vi "Server UI.vi"(11 "LV Chat Server in":refnum<class "LV Chat Server.lvclass">) -> (3 "LV Chat Server":refnum<class "LV Chat Server.lvclass">)   [LabVIEW 2020, in "LV Chat Server.lvclass"]
uses:
  LV Chat Server.lvclass
  UI State.ctl
  Data Types/Message.ctl
  LV Chat Server.lvclass/LV Chat Server.ctl
  Events.ctl
  Stream-Simple-Msg/Endpoint/Endpoint.lvclass
  Log Event Data.ctl
panel:
  in  "Timestamps":bool
  out "Time Connected":dbl format="%<%m/%d %H:%M:%S>T"
  out "Connection":string
  out "Users Connected":i32
  in  "Kick User":bool
  out "Log":string
  in  "Users":i32(listbox)
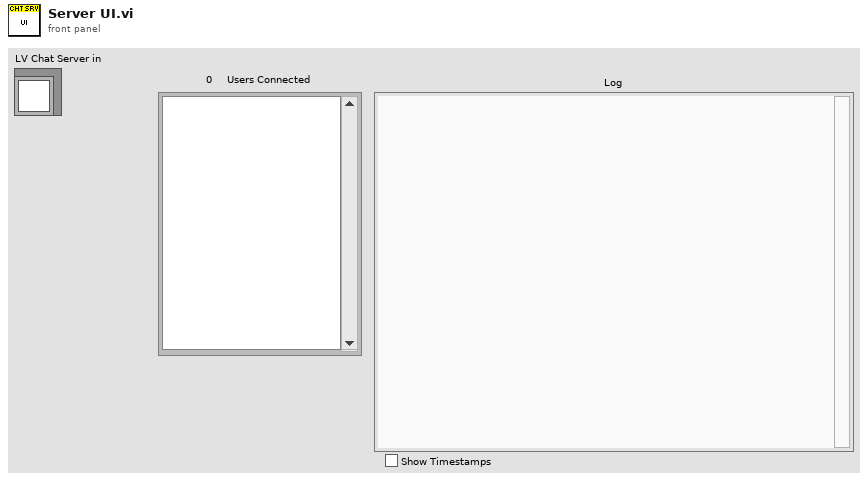
[diagram p1: front panel]
types:
  T1 = typedef "LV Chat Server.lvclass/UI State.ctl" = enum16{"Init", "Run", "Close"}
  T2 = typedef "Message.ctl" = cluster{"From":string, "Time":dbl, "Message":string}
  T3 = typedef "LV Chat Server.lvclass/Events.ctl" = cluster{"New Connection":refnum<user-event>, "Log":refnum<user-event>, "Refresh Log":refnum<user-event>, "Refresh Users":refnum<user-event>}
  T4 = typedef "LV Chat Server.lvclass/Ref Data.ctl" = cluster{"Endpoint Map":map{string, T5}, "User Map":map{string, string}}
  T5 = typedef "LV Chat Server.lvclass/User.ctl" = cluster{"Name":string, "IP":string, "Connected At":dbl, "Endpoint":refnum<class "Endpoint.lvclass">}
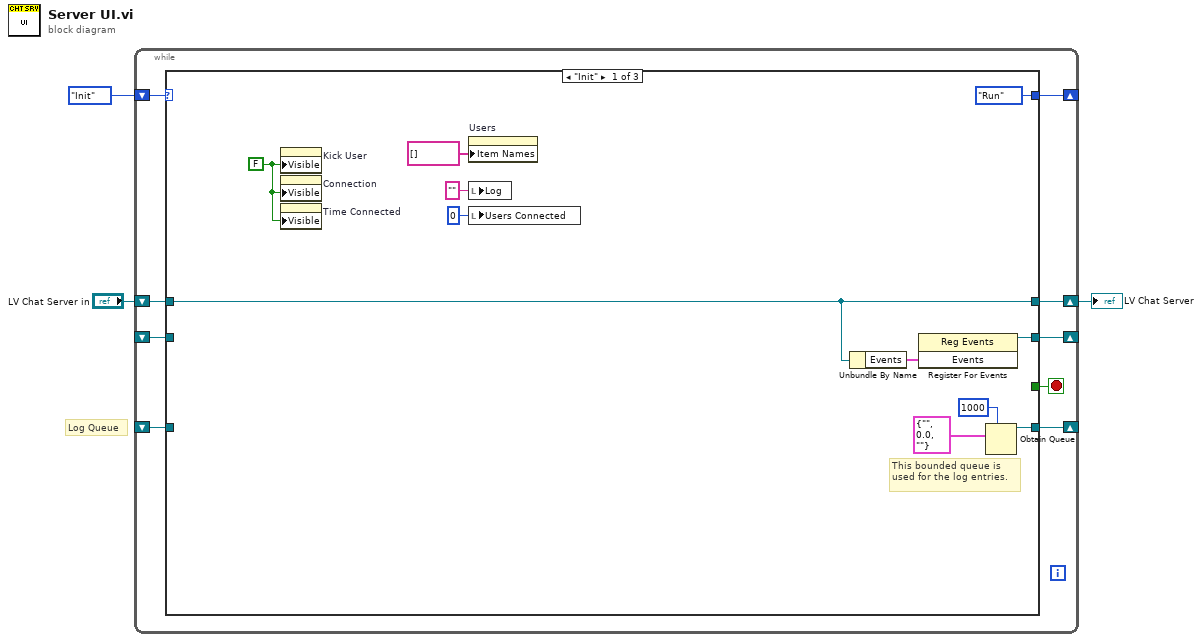
[diagram p0: block diagram]
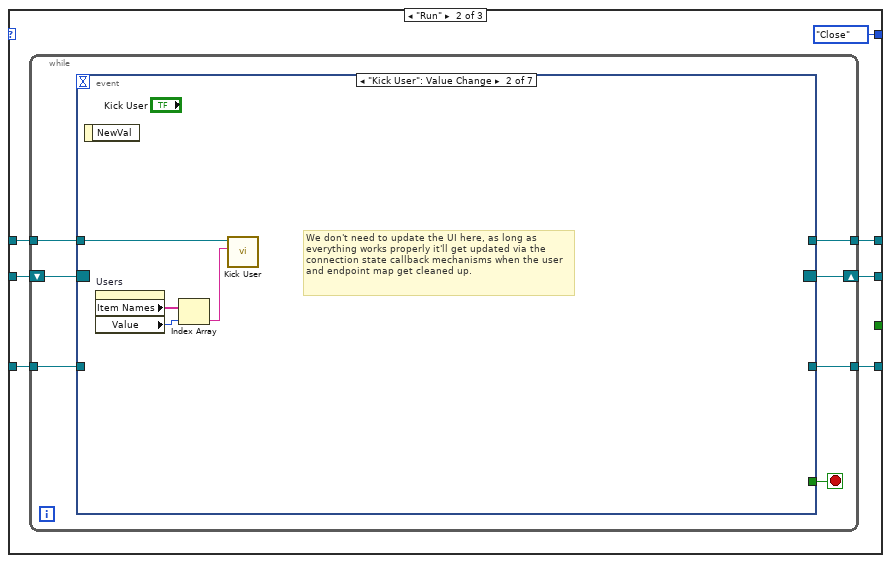
[diagram p2: hidden frame]
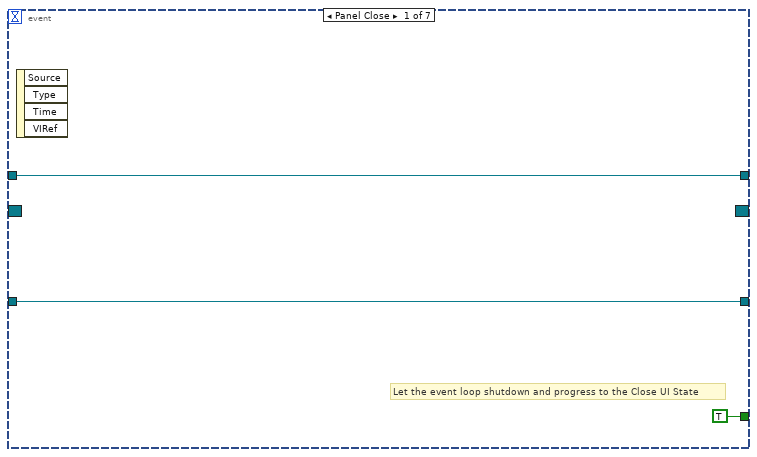
[diagram p3: hidden frame]
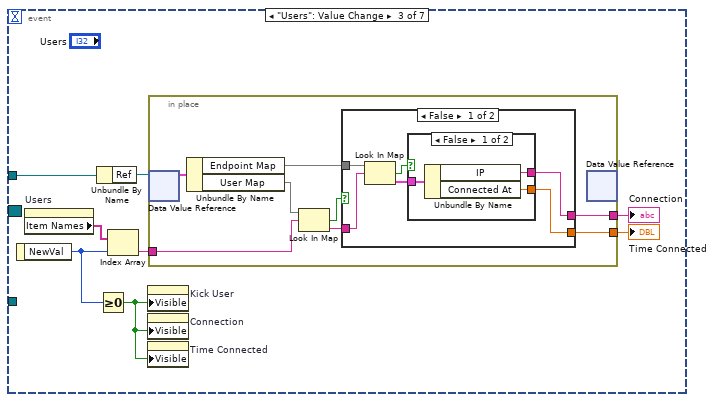
[diagram p4: hidden frame]
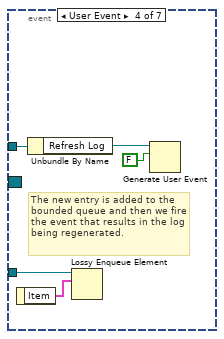
[diagram p7: hidden frame]
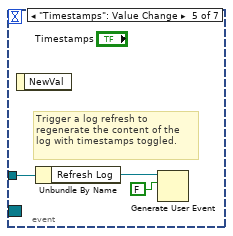
[diagram p8: hidden frame]
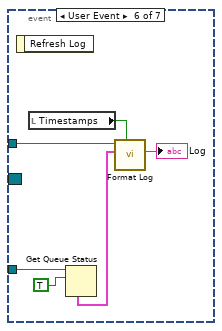
[diagram p9: hidden frame]
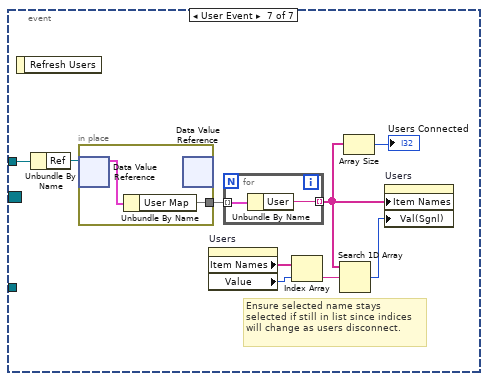
[diagram p10: hidden frame]
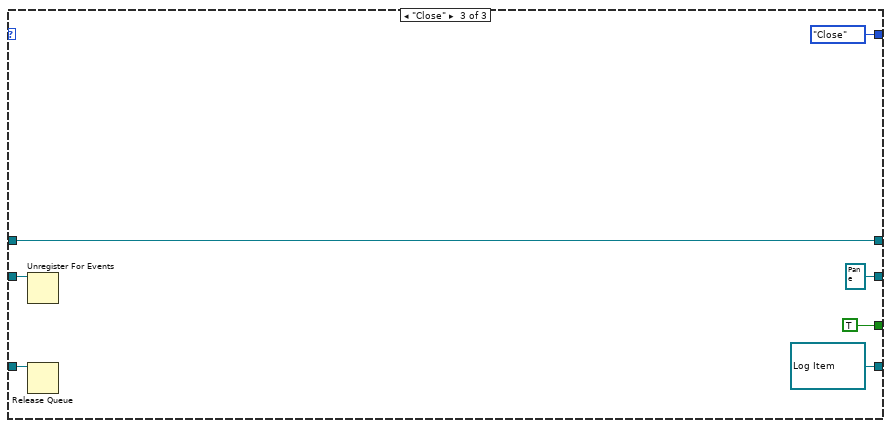
[diagram p11: hidden frame]
diagram:
  # "Log Queue"
  n1 = while {
    shift-right: [w11] -> w2
    shift-left: "LV Chat Server in" -> [w12]
    shift-right: [w9] -> _
    shift-left: _ -> [w8]
    shift-right: [w7] -> _
    shift-left: UI_State."Init" ("UI State") -> [w10]
    shift-right: [w5] -> _
    shift-left: _ -> [w4]
    stop <- w6 stop-if-true
    n2 = case shown="\"Init\"" w10 {
      tunnel: w12 -> [w21 w30 w101]
      tunnel: [w21 w29 w101] -> w11
      tunnel: [w20 w26 refnum<event-registration> refnum ("Event Registration Refnum")] -> w9
      tunnel: w8 -> [_ w28 w102]
      tunnel: [UI_State."Run" ("UI State") UI_State."Close" ("UI State") UI_State."Close" ("UI State")] -> w7
      tunnel: [_ _ TRUE] -> w6
      tunnel: [w16 w24 refnum<queue> refnum ("queue out")] -> w5
      tunnel: w4 -> [_ w25 w97]
      frame "Init" {
        w15 = FALSE ("Visible")
        # "This bounded queue is used for the log entries."
        n3 = property on="Kick User" class="Bool"("Visible"=w15) -> ()  [unwired: 2 in, 2 out]
        n4 = property on="Connection" class="Str"("Visible"=w15) -> ()  [unwired: 2 in, 2 out]
        n5 = property on="Time Connected" class="DigNum (strict)"("Visible"=w15) -> ()  [unwired: 2 in, 2 out]
        n6 = property on="Users" class="LstBox (strict)"("Item Names"=string[] []) -> ()  [unwired: 2 in, 2 out]
        n7 = local write "Log"("" ("Log")) -> ()
        n8 = local write "Users Connected"(0 ("Users Connected")) -> ()
        n9 = Unbundle By Name(w21) -> ("Events"=w22:T3)
        n10 = register-events(w22) -> (reference out=w20:refnum<event-registration>)  [unwired: 2 in, 1 out]
        n11 = Obtain Queue(max queue size (-1, unlimited)=1000, element data type=T2 {"From"="", "Time"=0.0, "Message"=""} ("Log Item")) -> (queue out=w16:refnum<queue>)  [unwired: 3 in, 2 out]
      }
      frame "Run" {
        n12 = while {
          tunnel: w30 -> [w36]
          tunnel: [w35] -> w29
          shift-right: [w33] -> w26
          shift-left: w28 -> [w34]
          tunnel: w25 -> [w32]
          tunnel: [w31] -> w24
          stop <- w37 stop-if-true
          n13 = event shown="[1] \"Kick User\": Value Change" {
            selector: w34 -> [_ _ _ _ _ _ _]
            dyn-events: [_ _ _ _ _ _ _] -> w33
            timeout: _ -> [_ _ _ _ _ _ _]
            tunnel: [TRUE _ _ _ _ _ _] -> w37
            tunnel: w36 -> [w39 w42 w50 w70 w77 w81 w91]
            tunnel: [w39 _ _ _ _ _ _] -> w35
            tunnel: w32 -> [w38 _ _ w74 _ w83 _]
            tunnel: [w38 _ _ _ _ _ _] -> w31
            event Panel Close {
              # "Let the event loop shutdown and progress to the Close UI State"
              n14 = event-data() -> ()  [unwired: 1 in, 4 out]
            }
            event "Kick User": Value Change {
              # "We don't need to update the UI here, as long as everything works properly it'll get updated via the connection state callback mechanisms when the user and endpoint map get cleaned up."
              n15 = event-data() -> ()  [unwired: 1 in, 1 out]
              n16 = property on="Users" class="LstBox (strict)"() -> ("Item Names"=w44:string[], "Value"=w43:i32)  [unwired: 2 in, 2 out]
              n17 = Index Array(array=w44, index=w43) -> (element=w41:string)
              n18 = call "Kick User.vi"("User"=w41, "LV Chat Server in"=w42) -> ()  [unwired: 8 in, 2 out]
            }
            event "Users": Value Change {
              n19 = event-data() -> ("NewVal"=w47:i32)  [unwired: 1 in]
              n20 = property on="Users" class="LstBox (strict)"() -> ("Item Names"=w52:string[])  [unwired: 2 in, 2 out]
              n21 = Unbundle By Name(w50) -> ("Ref"=w51:refnum<data-value>)
              n22 = Greater Or Equal To 0?(x=w47) -> (x >= 0?=w45:bool)
              n23 = Index Array(array=w52, index=w47) -> (element=w49:string)
              n24 = property on="Kick User" class="Bool"("Visible"=w45) -> ()  [unwired: 2 in, 2 out]
              n25 = property on="Connection" class="Str"("Visible"=w45) -> ()  [unwired: 2 in, 2 out]
              n26 = property on="Time Connected" class="DigNum (strict)"("Visible"=w45) -> ()  [unwired: 2 in, 2 out]
              n27 = in-place {
                in-place-border: w49 -> [w58]
                in-place-border: [w54] -> w48
                in-place-border: [w53] -> w46
                n28 = in-place-dvr #1(w51) -> (w60:T4)  [unwired: 1 out]
                n29 = Unbundle By Name(w60) -> ("Endpoint Map"=w55:map{string, T5}, "User Map"=w59:map{string, string})
                n30 = Look In Map(map=w59, key=w58) -> (key not found?=w57:bool, value=w56:string)  [unwired: 1 in]
                n31 = case shown="False" w57 {
                  tunnel: w56 -> [w65 _]
                  tunnel: w55 -> [w66 _]
                  tunnel: [w63 _] -> w54
                  tunnel: [w62 _] -> w53
                  frame False {
                    n32 = Look In Map(map=w66, key=w65) -> (key not found?=w61:bool, value=w64:T5)  [unwired: 1 in]
                    n33 = case shown="False" w61 {
                      tunnel: w64 -> [w69 _]
                      tunnel: [w68 _] -> w63
                      tunnel: [w67 _] -> w62
                      frame False {
                        n34 = Unbundle By Name(w69) -> ("IP"=w68:string, "Connected At"=w67:dbl)
                      }
                      frame True {
                      }
                    }
                  }
                  frame True {
                  }
                }
                n35 = in-place-dvr #1() -> ()  [unwired: 1 in, 2 out]
              }
              "Connection" <- w48
              "Time Connected" <- w46
            }
            event User Event {
              # "The new entry is added to the bounded queue and then we fire the event that results in the log being regenerated."
              n36 = event-data() -> ("Item"=w73:T2)  [unwired: 1 in]
              n37 = Unbundle By Name(w70) -> ("Refresh Log"=w72:refnum<user-event>)
              n38 = Lossy Enqueue Element(queue=w74, element=w73) -> ()  [unwired: 1 in, 4 out]
              n39 = Generate User Event(user event=w72, event data cluster=FALSE ("event data")) -> ()  [unwired: 2 in, 2 out]
            }
            event "Timestamps": Value Change {
              # "Trigger a log refresh to regenerate the content of the log with timestamps toggled."
              n40 = event-data() -> ()  [unwired: 1 in, 1 out]
              n41 = Unbundle By Name(w77) -> ("Refresh Log"=w76:refnum<user-event>)
              n42 = Generate User Event(user event=w76, event data cluster=FALSE ("event data")) -> ()  [unwired: 2 in, 2 out]
            }
            event User Event {
              n43 = event-data() -> ()  [unwired: 1 in, 1 out]
              n44 = local read "Timestamps"() -> (w79:bool)
              n45 = Get Queue Status(queue=w83, return elements? (F)=TRUE) -> (elements=w80:T2[])  [unwired: 1 in, 7 out]
              n46 = call "Format Log.vi"("Timestamps"=w79, "Items"=w80, "LV Chat Server in"=w81) -> ("Log"=→"Log":string)  [unwired: 6 in, 2 out]
            }
            event User Event {
              # "Ensure selected name stays selected if still in list since indices will change as users disconnect."
              n47 = event-data() -> ()  [unwired: 1 in, 1 out]
              n48 = Unbundle By Name(w91) -> ("Ref"=w92:refnum<data-value>)
              n49 = in-place {
                in-place-border: [w95] -> w90
                n50 = in-place-dvr #2(w92) -> (w96:T4)  [unwired: 1 out]
                n51 = Unbundle By Name(w96) -> ("User Map"=w95:map{string, string})
                n52 = in-place-dvr #2() -> ()  [unwired: 1 in, 2 out]
              }
              n53 = property on="Users" class="LstBox (strict)"() -> ("Item Names"=w89:string[], "Value"=w88:i32)  [unwired: 2 in, 2 out]
              n54 = for {
                tunnel: w90 -> [w94] mode=indexing
                tunnel: [w93] -> w85 mode=indexing
                n55 = Unbundle By Name(w94) -> ("User"=w93:string)
              }
              n56 = Index Array(array=w89, index=w88) -> (element=w87:string)
              n57 = Search 1D Array(1D array=w85, element=w87) -> (index of element=w86:i32)  [unwired: 1 in]
              n58 = Array Size(array=w85) -> (size(s)=→"Users Connected":i32)
              n59 = property on="Users" class="LstBox (strict)"("Item Names"=w85, "Val(Sgnl)"=w86) -> ()  [unwired: 2 in, 2 out]
            }
          }
        }
      }
      frame "Close" {
        n60 = Unregister For Events(event registration refnum=w102) -> ()  [unwired: 1 in, 1 out]
        n61 = Release Queue(queue=w97) -> ()  [unwired: 2 in, 3 out]
      }
    }
  }
  "LV Chat Server" <- w2
